vi "applyInsertSpaceY.vi"(4 "deltaY":u16, 8 "error in (no error)":errorcluster, 10 "originY":i32, 11 "AbstractDiagram in":refnum<class "AbstractDiagram.lvclass">) -> (0 "error out":errorcluster, 3 "AbstractDiagram out":refnum<class "AbstractDiagram.lvclass">)   [LabVIEW 2023, in "TLC_Scripto.lvlib" / "AbstractDiagram.lvclass"]
uses:
  AbstractDiagram.lvclass
  AbstractDiagram.lvclass/AbstractDiagram.ctl
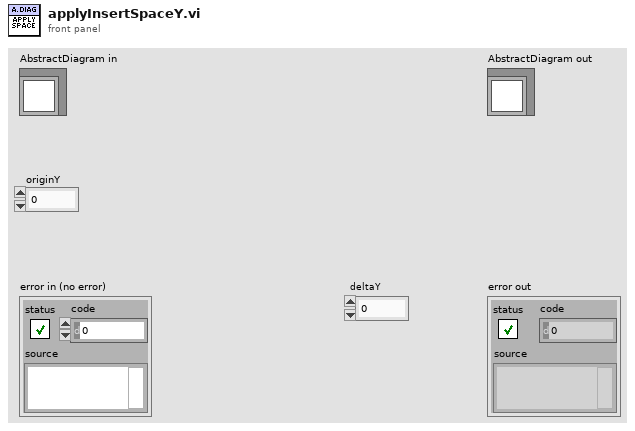
[diagram p1: front panel]
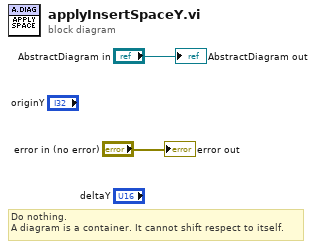
[diagram p0: block diagram]
diagram:
  # "Do nothing.\nA diagram is a container. It cannot shift respect to itself."
  "error out" <- "error in (no error)"
  "AbstractDiagram out" <- "AbstractDiagram in"
